vi "Get Node Children Data RecursiveChild.vi"(10 "Node Path (parent, child)":string[](array[string]), 11 "Tree Map In":T4) -> (0 "error out":errorcluster, 1 "Node Exists?":bool, 2 "tree node data map":T1, 3 "Tree Map Out":T4)   [LabVIEW 2020, in "Blue Tree Map OpenSource.lvlib"]
uses:
  Blue Tree Map OpenSource.lvlib
  Typedefs/Tree Map.ctl
  Typedefs/Tree Map Data.ctl
  Typedefs/Tree Node Data.ctl
  Typedefs/Attribute Map.ctl
  Typedefs/Tree Node Data Map.ctl
  <vilib>/Utility/miscctls.llb/LVMapReplaceAction.ctl
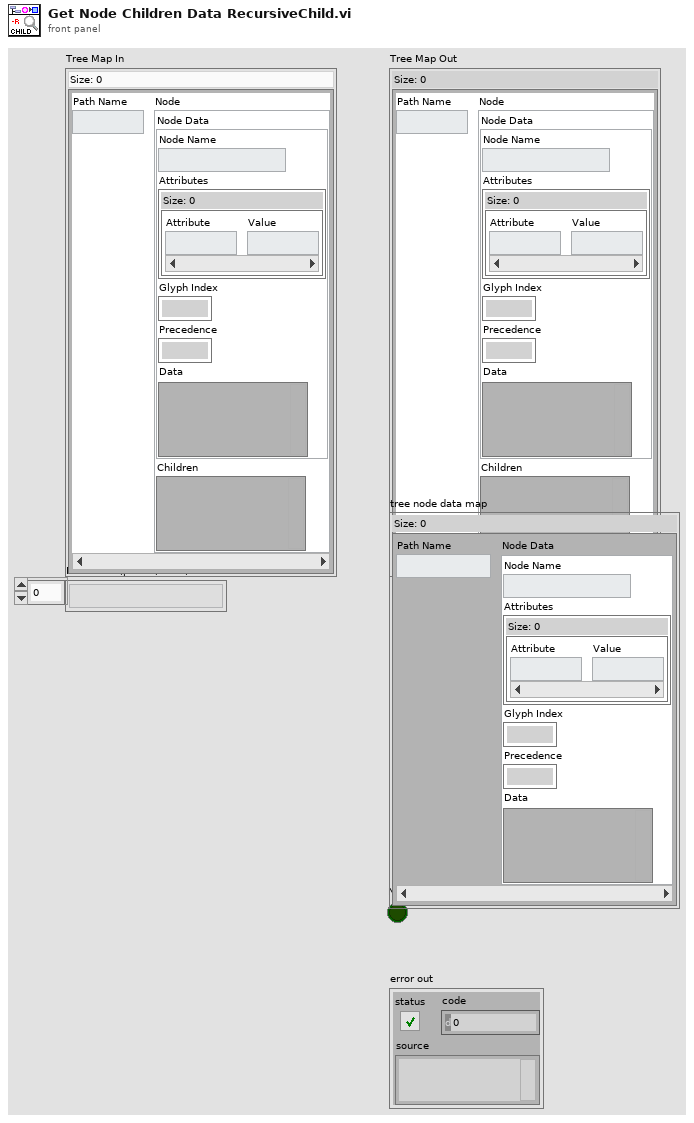
[diagram p1: front panel]
types:
  T1 = typedef "Blue Tree Map OpenSource.lvlib/Tree Node Data Map.ctl" = map{string, T2}
  T2 = typedef "Blue Tree Map OpenSource.lvlib/Tree Node Data.ctl" = cluster{"Node Name":string, "Attributes":T3, "Glyph Index":i32, "Precedence":i32, "Data":variant}
  T3 = typedef "Blue Tree Map OpenSource.lvlib/Attribute Map.ctl" = map{string, string}
  T4 = typedef "Blue Tree Map OpenSource.lvlib/Tree Map.ctl" = map{string, T5}
  T5 = typedef "Blue Tree Map OpenSource.lvlib/Tree Map Data.ctl" = cluster{"Node Data":T2, "Children":variant}
  T6 = typedef "LVMapReplaceAction.ctl" = enum32{"Modify Entry only if found", "Add or Modify Entry", "Delete Entry"}
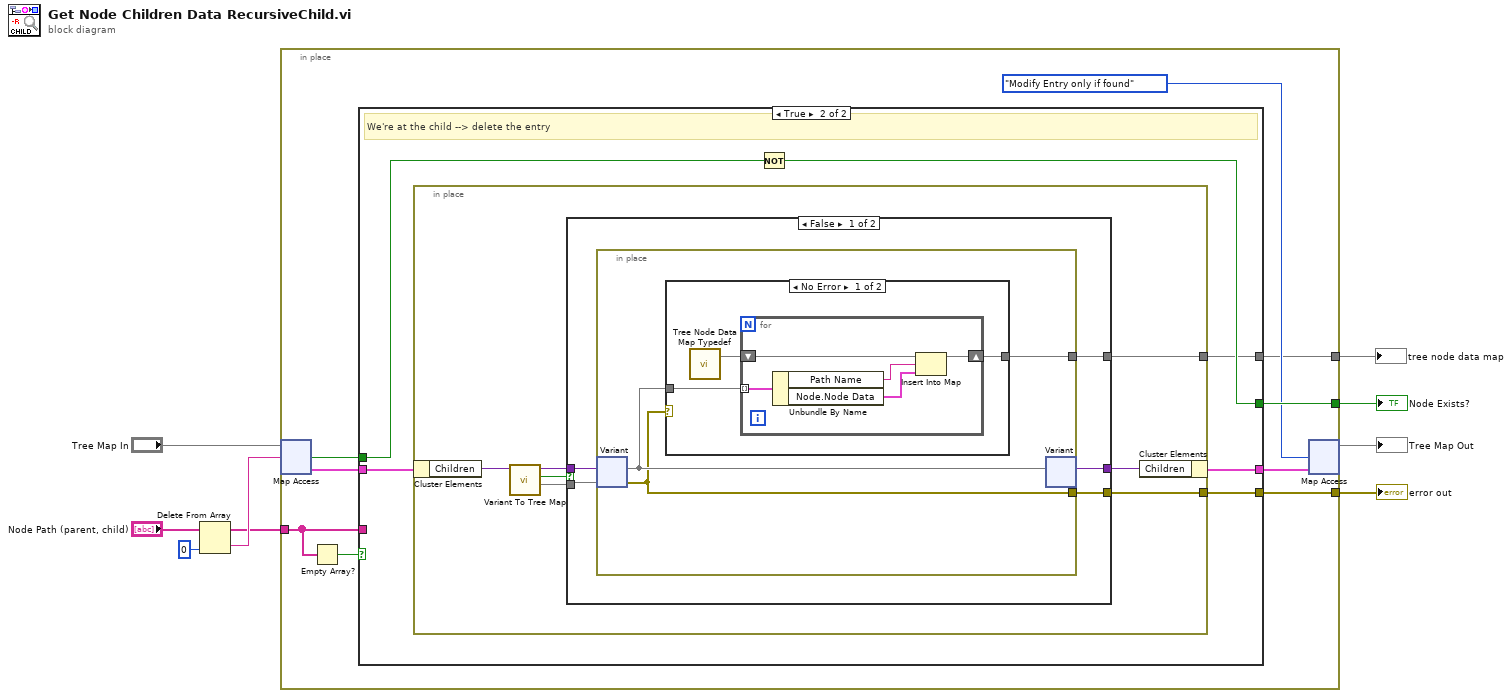
[diagram p0: block diagram]
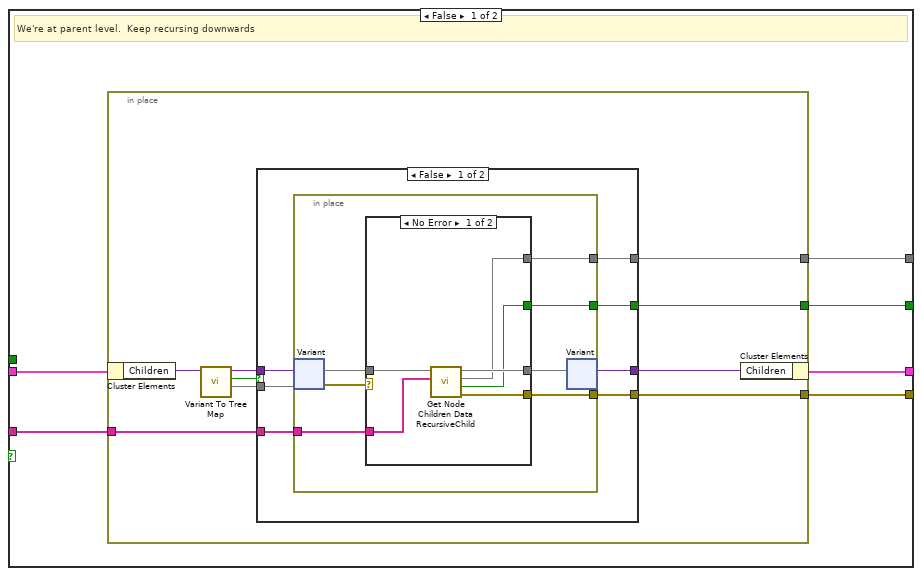
[diagram p2: hidden frame]
diagram:
  n1 = Delete From Array(array="Node Path (parent, child)", index=0) -> (deleted portion=w8:string, array with subset deleted=w7:string[])  [unwired: 1 in]
  n2 = in-place {
    in-place-border: w7 -> [w12]
    in-place-border: [w17] -> w3
    in-place-border: [w15] -> w4
    in-place-border: [w10] -> w1
    n3 = in-place-map #1("Tree Map In", w8) -> (w18:T5, w14:bool)  [unwired: 1 in]
    n4 = Empty Array?(array=w12) -> (empty?=w13:bool)
    n5 = case shown="True" w13 {
      tunnel: w18 -> [w24 w60]
      tunnel: w12 -> [w23 _]
      tunnel: [w22 w57] -> w17
      tunnel: [w21 w59] -> w16
      tunnel: [w20 w62] -> w15
      tunnel: w14 -> [_ w61]
      tunnel: [w19 w58] -> w10
      frame False {
        # "We're at parent level.  Keep recursing downwards"
        n6 = in-place {
          in-place-border: w23 -> [w32]
          in-place-border: [w31] -> w22
          in-place-border: [w30] -> w20
          in-place-border: [w25] -> w19
          n7 = in-place-cluster #2(w24) -> ("Children"=w33:variant)
          n8 = call "Variant To Tree Map.vi"("Children"=w33) -> ("Tree Map (Empty)"=w28:T4, "Empty?"=w27:bool, "Children"=w29:variant)  [unwired: 8 in]
          n9 = case shown="False" w27 {
            tunnel: w32 -> [w40 _]
            tunnel: [w39 _] -> w31
            tunnel: [w38 _] -> w30
            tunnel: w29 -> [w37 w56]
            tunnel: w28 -> [w36 _]
            tunnel: [w35 w56] -> w26
            tunnel: [w34 _] -> w25
            frame False {
              n10 = in-place {
                in-place-border: w40 -> [w47]
                in-place-border: [w46] -> w39
                in-place-border: [w45] -> w38
                in-place-border: [w41] -> w34
                n11 = in-place-variant #3(w37, w36) -> (w44:T4, w42:errorcluster)
                n12 = case shown="No Error" w42 {
                  selector: w42 -> [_ w54]
                  tunnel: w47 -> [w50 _]
                  tunnel: [w51 w54] -> w46
                  tunnel: [w49 _] -> w45
                  tunnel: w44 -> [w53 w55]
                  tunnel: [w52 w55] -> w43
                  tunnel: [w48 _] -> w41
                  frame No Error {
                    n13 = call "Get Node Children Data RecursiveChild.vi"("Node Path (parent, child)"=w50, "Tree Map In"=w53) -> ("error out"=w51:errorcluster, "Node Exists?"=w49:bool, "tree node data map"=w48:T1, "Tree Map Out"=w52:T4)  [unwired: 6 in]
                  }
                  frame Error {
                  }
                }
                n14 = in-place-variant #3(w43) -> (w35:variant)  [unwired: 1 out]
              }
            }
            frame True {
            }
          }
          n15 = in-place-cluster #2("Children"=w26) -> (w21:T5)
        }
      }
      frame True {
        # "We're at the child --> delete the entry"
        n16 = in-place {
          in-place-border: [w64] -> w58
          in-place-border: [w63] -> w57
          n17 = in-place-cluster #4(w60) -> ("Children"=w69:variant)
          n18 = call "Variant To Tree Map.vi"("Children"=w69) -> ("Tree Map (Empty)"=w66:T4, "Empty?"=w68:bool, "Children"=w67:variant)  [unwired: 8 in]
          n19 = case shown="False" w68 {
            tunnel: w67 -> [w74 w86]
            tunnel: w66 -> [w73 _]
            tunnel: [w72 w86] -> w65
            tunnel: [w71 _] -> w64
            tunnel: [w70 _] -> w63
            frame False {
              n20 = in-place {
                in-place-border: [w76] -> w71
                in-place-border: [w75] -> w70
                n21 = in-place-variant #5(w74, w73) -> (w77:T4, w75:errorcluster)
                n22 = case shown="No Error" w75 {
                  tunnel: w77 -> [w80 _]
                  tunnel: [w78 _] -> w76
                  frame No Error {
                    n23 = call "Tree Node Data Map Typedef.vi"() -> ("tree node data map"=w79:T1)  [unwired: 3 in]
                    n24 = for {
                      tunnel: w80 -> [w85] mode=indexing
                      shift-right: [w81] -> w78
                      shift-left: w79 -> [w84]
                      n25 = Unbundle By Name(w85) -> ("Path Name"=w83:string, "Node.Node Data"=w82:T2)
                      n26 = Insert Into Map(map in=w84, key=w83, value=w82) -> (map out=w81:T1)  [unwired: 2 out]
                    }
                  }
                  frame Error {
                  }
                }
                n27 = in-place-variant #5(w77) -> (w72:variant)  [unwired: 1 out]
              }
            }
            frame True {
            }
          }
          n28 = in-place-cluster #4("Children"=w65) -> (w59:T5)
        }
        n29 = Not(x=w61) -> (.not. x?=w62:bool)
      }
    }
    n30 = in-place-map #1(w16, LVMapReplaceAction."Modify Entry only if found" ("action")) -> (→"Tree Map Out":T4)  [unwired: 2 out]
  }
  "error out" <- w3
  "Node Exists?" <- w4
  "tree node data map" <- w1
